vi "Read Roles.vi"(8 "error in (no error)":errorcluster, 11 "PassPlay in":refnum<class "PassPlay.lvclass">) -> (0 "error out":errorcluster, 2 "Roles":T1, 3 "PassPlay out":refnum<class "PassPlay.lvclass">)   [LabVIEW 2024, in "PassPlay.lvclass"]
uses:
  PassPlay.lvclass
  PassKickerRole_class/PassKickerRole.lvclass
  PassReceiverRole_class/PassReceiverRole.lvclass
  PassPlay.lvclass/PassPlay.ctl
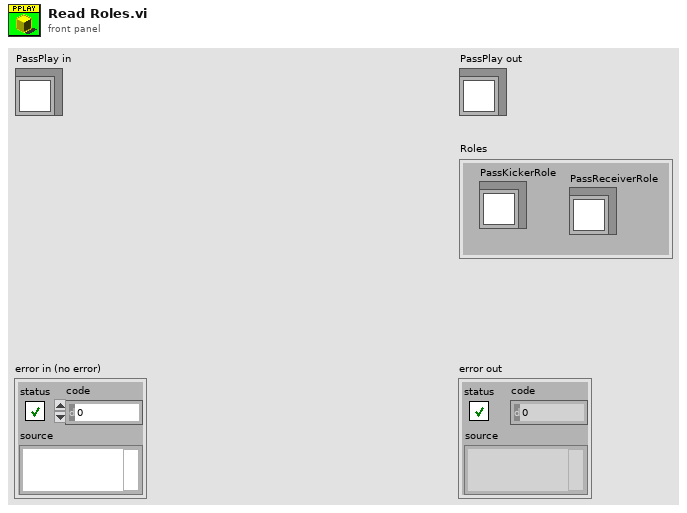
[diagram p1: front panel]
types:
  T1 = cluster{"PassKickerRole":refnum<class "PassKickerRole.lvclass">, "PassReceiverRole":refnum<class "PassReceiverRole.lvclass">}
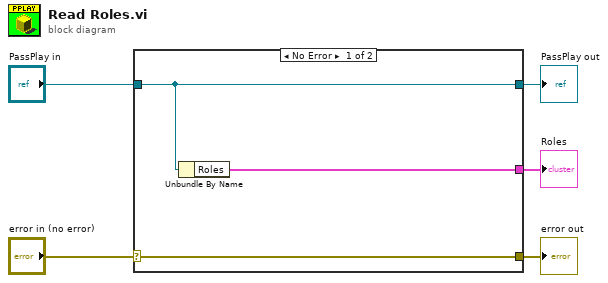
[diagram p0: block diagram]
diagram:
  n1 = case shown="No Error" "error in (no error)" {
    selector: "error in (no error)" -> [w8 w9]
    tunnel: [w8 w9] -> w4
    tunnel: [w7 w10] -> w2
    tunnel: "PassPlay in" -> [w7 w10]
    tunnel: [w6 _] -> w1
    frame No Error {
      n2 = Unbundle By Name(w7) -> ("Roles"=w6:T1)
    }
    frame Error {
    }
  }
  "error out" <- w4
  "PassPlay out" <- w2
  "Roles" <- w1
